vi "PXI-4130 Updated Channels (RT).vi"(5 "Channel Type":T1 items=["Voltage Controlled", "Current Controlled"], 7 "Channel":string, 8 "error in (no error)":errorcluster, 10 "Data In":dbl[](array[numeric]), 11 "resource name In":refnum<k15>) -> (0 "error out":errorcluster, 2 "Data Out":dbl[](array[numeric]), 3 "resource name Out":refnum<k15>)   [LabVIEW 2009, in "PXI-4130 Custom Device.lvlib"]
uses:
  PXI-4130 Custom Device.lvlib
  Channel Type.ctl
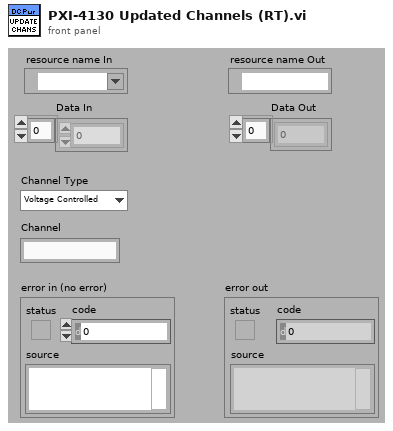
[diagram p1: front panel]
types:
  T1 = typedef "PXI-4130 Custom Device.lvlib/Channel Type.ctl" = i32
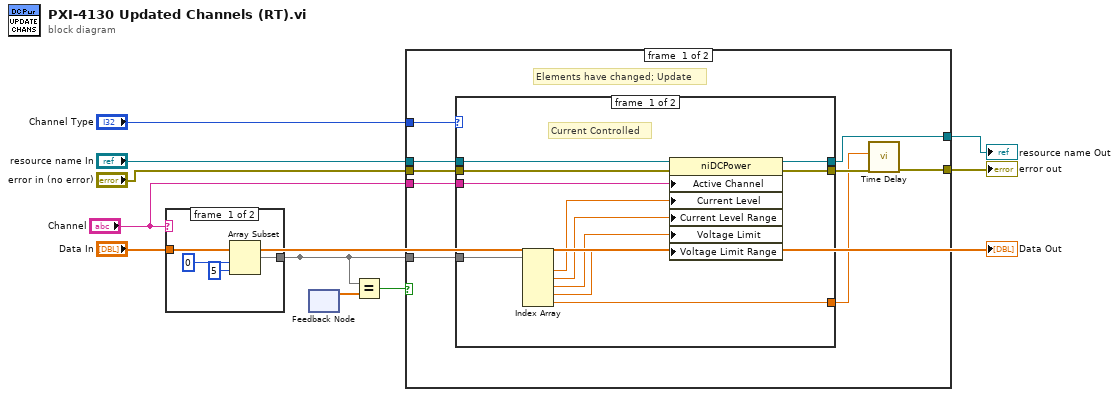
[diagram p0: block diagram]
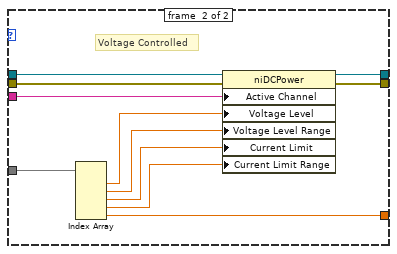
[diagram p2: hidden frame]
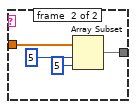
[diagram p4: hidden frame]
diagram:
  n1 = case shown="\"0\", Default" "Channel" {
    tunnel: "Data In" -> [w14 w18]
    tunnel: [w11 w15] -> w2
    frame #0 {
      n2 = Array Subset(array=w14, index=0, length=5) -> (w11:dbl[])
    }
    frame #1 {
      n3 = Array Subset(array=w18, index=5, length=5) -> (w15:dbl[])
    }
  }
  n4 = feedback #1() -> (w3:dbl[])  [unwired: 1 in]
  n5 = Equal?(x=w2, y=w3) -> (x = y?=w1:bool)
  n6 = case shown="False" w1 {
    tunnel: w2 -> [w27 _]
    tunnel: "Channel Type" -> [w26 _]
    tunnel: [w23 w50] -> w9
    tunnel: [w22 w51] -> w7
    tunnel: "Channel" -> [w21 _]
    tunnel: "resource name In" -> [w20 w51]
    tunnel: "error in (no error)" -> [w19 w50]
    frame #0 {
      # "Elements have changed; Update"
      n7 = case shown="0, Default" w26 {
        tunnel: w20 -> [w38 w49]
        tunnel: w27 -> [w37 w48]
        tunnel: [w33 w44] -> w22
        tunnel: [w32 w43] -> w25
        tunnel: [w31 w42] -> w24
        tunnel: w19 -> [w30 w41]
        tunnel: w21 -> [w28 w39]
        frame #0 {
          # "Current Controlled"
          n8 = Index Array(array=w37) -> (element #1=w29:dbl, element #2=w36:dbl, element #3=w35:dbl, element #4=w34:dbl, element #5=w31:dbl)  [unwired: 5 in]
          n9 = property class="niDCPower"(reference=w38, error in=w30, "Active Channel"=w28, "Current Level"=w29, "Current Level Range"=w36, "Voltage Limit"=w35, "Voltage Limit Range"=w34) -> (reference out=w33:refnum<k15>, error out=w32:errorcluster)
        }
        frame #1 {
          # "Voltage Controlled"
          n10 = Index Array(array=w48) -> (element #1=w40:dbl, element #2=w47:dbl, element #3=w46:dbl, element #4=w45:dbl, element #5=w42:dbl)  [unwired: 5 in]
          n11 = property class="niDCPower"(reference=w49, error in=w41, "Active Channel"=w39, "Voltage Level"=w40, "Voltage Level Range"=w47, "Current Limit"=w46, "Current Limit Range"=w45) -> (reference out=w44:refnum<k15>, error out=w43:errorcluster)
        }
      }
      n12 = call "Time Delay"("error in (no error)"=w25, "Delay Time (s)"=w24) -> ("error out"=w23:errorcluster)  [unwired: 9 in]
    }
    frame #1 {
      # "Same as last iteration; Do nothing"
    }
  }
  "resource name Out" <- w7
  "error out" <- w9
  "Data Out" <- "Data In"
